vi "main_RL.vi"() -> ()   [LabVIEW 2017]
panel:
  in  "Tab Control":enum32{"Page 1", "Page 2"}(tab)
  in  "Next Button":bool
  out "Heater ON/OFF":bool caption="Heater"
  out "Pump ON/OFF":bool caption="Pump"
  in  "F1_F3":bool
  in  "T1_T3":bool
  out "NI1":tag caption="NI device"
  in  "Exit":bool
  in  "Tab Control 4":enum32{"Charts", "Diagram"}(tab)
  in  "Save as image 6":bool
  in  "Save as Excel 6":bool
  in  "Pause Button 6":bool
  in  "Reset Chart 6":bool
  in  "Save as image 5":bool
  in  "Save as Excel 5":bool
  in  "Pause Button 5":bool
  in  "Reset Chart 5":bool
  in  "Tab Control 2":enum32{"Page 1", "Page 2"}(tab)
  in  "Save as image 3":bool
  in  "Save as Excel 3":bool
  in  "Pause Button 3":bool
  in  "Reset Chart 3":bool
  out "T1 chart":dbl(graph)
  in  "Reset Chart":bool
  in  "Pause Button":bool
  in  "Save as Excel":bool
  in  "Save as image":bool
  out "T3 chart":dbl(graph)
  out "T2 chart":dbl(graph)
  out "F2 chart":dbl(graph)
  in  "Tab Control 3":enum32{"Page 1", "Page 2"}(tab)
  in  "Reset Chart 4":bool
  in  "Pause Button 4":bool
  in  "Save as Excel 4":bool
  in  "Save as image 4":bool
  out "F1 chart":dbl(graph)
  in  "Reset Chart 2":bool
  in  "Pause Button 2":bool
  in  "Save as Excel 2":bool
  in  "Save as image 2":bool
  out "F3 chart":dbl(graph)
  out "Heater":bool
  out "FlowMeter 3":bool
  out "FlowMeter 2":bool
  out "Pump":bool
  out "FlowMeter":bool
  out "T1":dbl format="%#.3f"
  out "T3":dbl format="%#_3f"
  out "F1":dbl format="%#.3f"
  out "F3":dbl format="%#_3f"
  out "T2":dbl format="%#.3f"
  out "F2":dbl format="%#.3f"
  in  "Pump 2":bool
  in  "Heater ON/OFF 2":bool
  # "Recycle Loops Unit"
  # "Cold Water Supply"
  # "To Drain"
  # "Water Heater"
  # "Water Filter"
  # "Pressure reducing valve"
  # "Pump"
  # "Throttling Valve"
  # "Temperature Sensor\n(T2)"
  # "Flow meter\n(F3)"
  # "Flow meter\n(F1)"
  # "Flow meter\n(F2)"
  # "Temperature Sensor\n(T1)"
  # "Temperature Sensor\n(T3)"
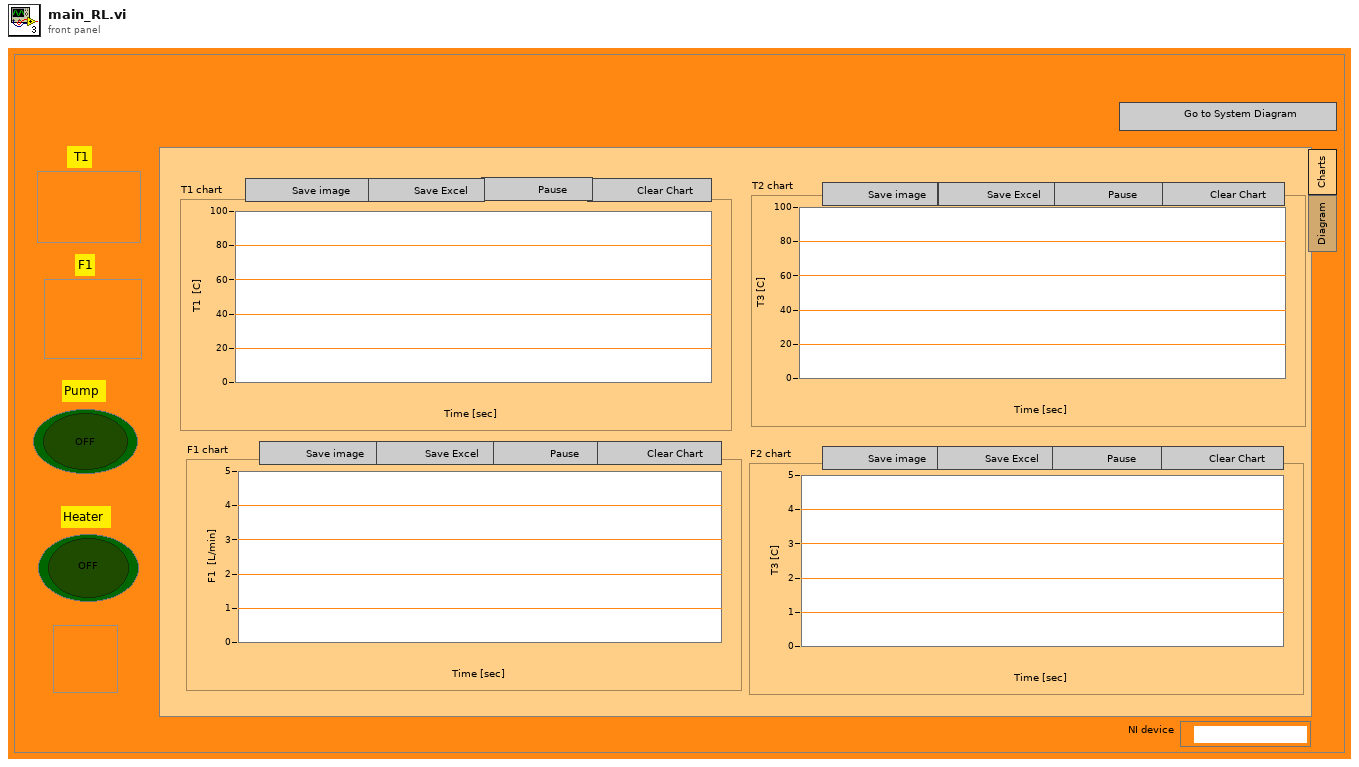
[diagram p1: front panel]
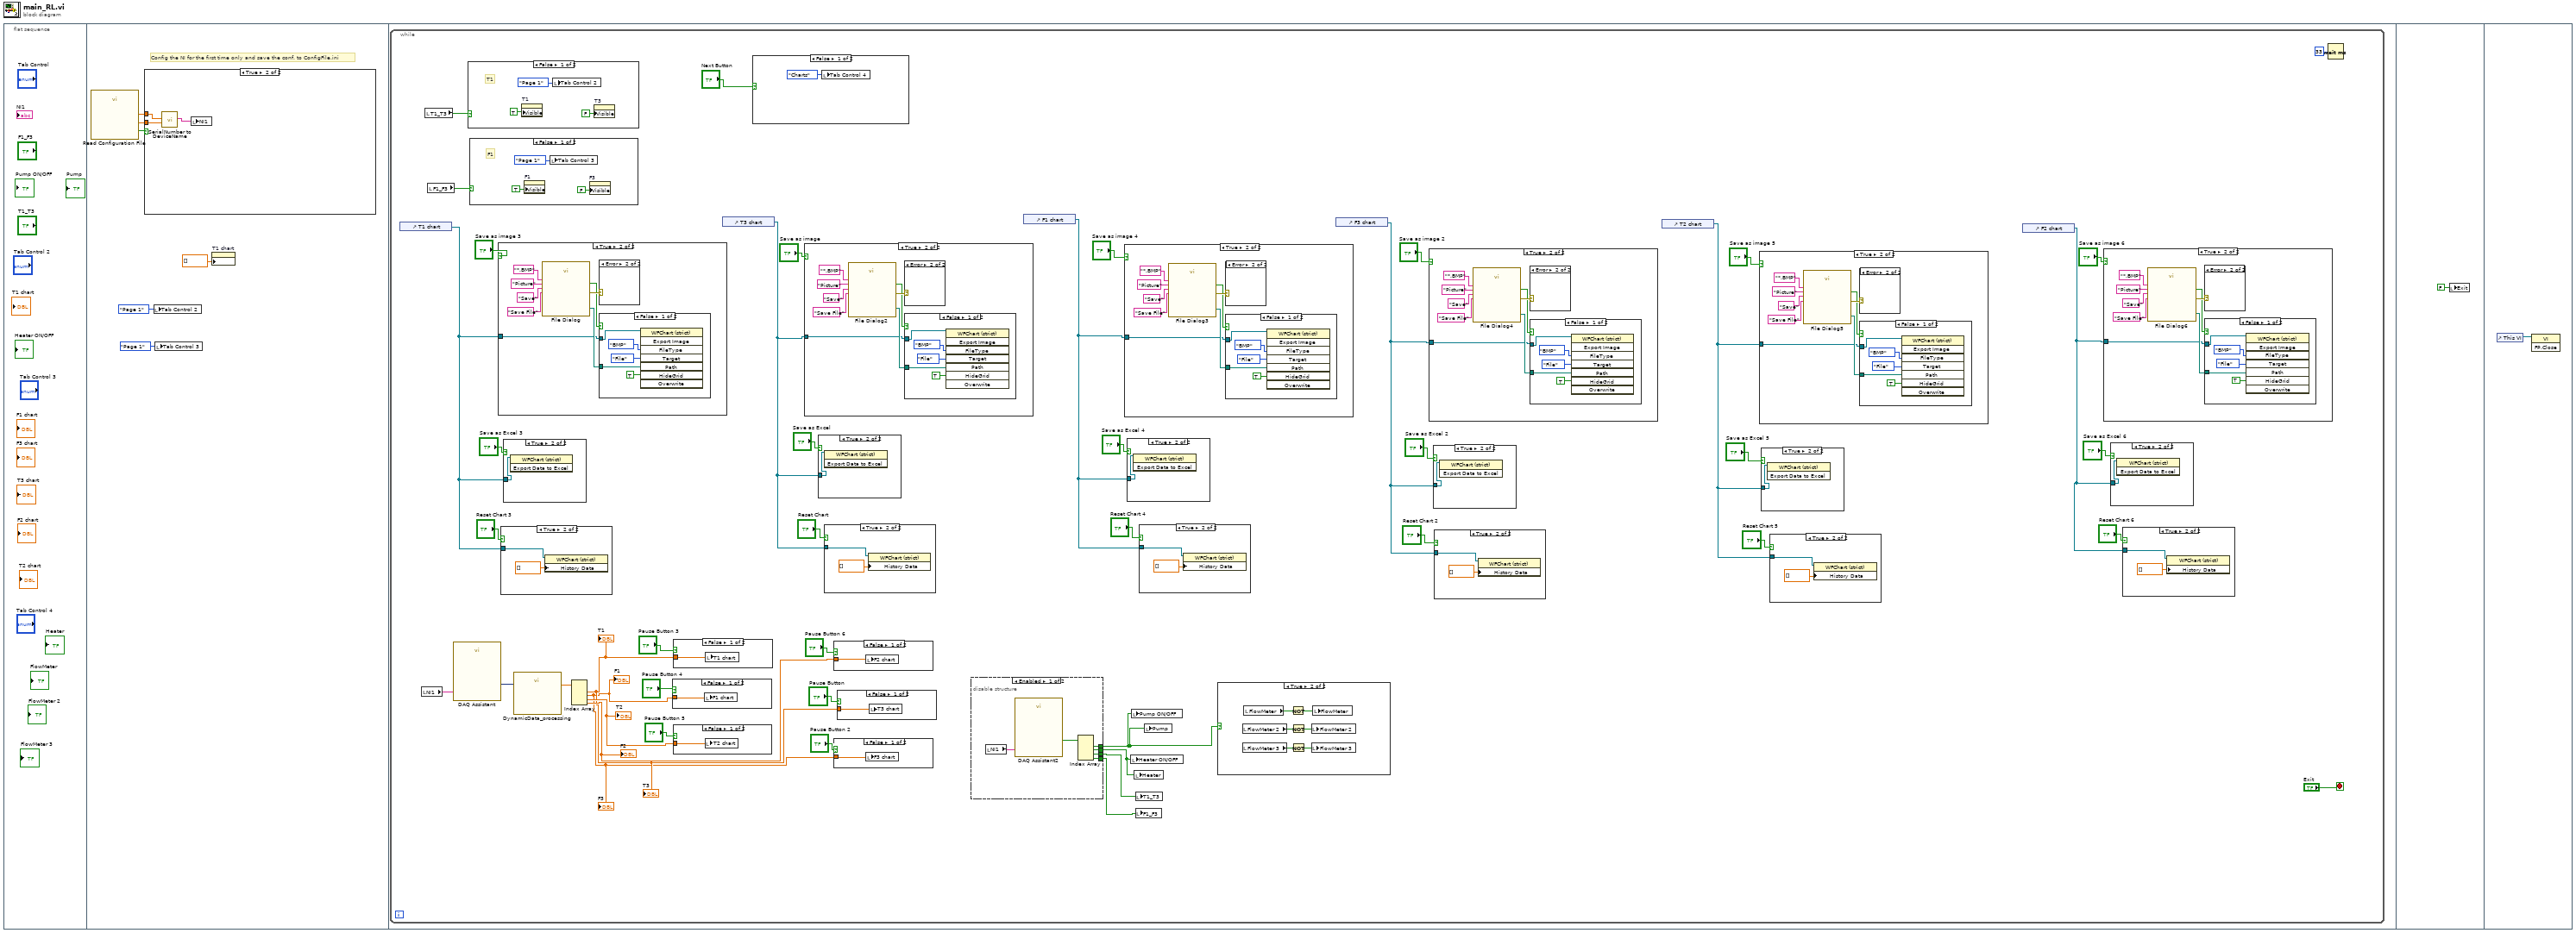
[diagram p0: block diagram]
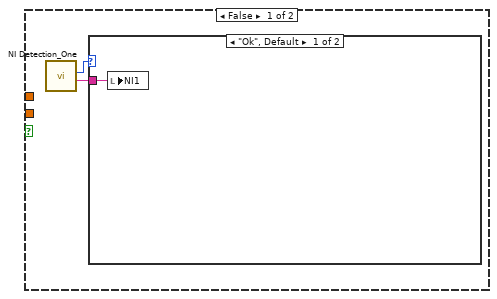
[diagram p2: hidden frame]
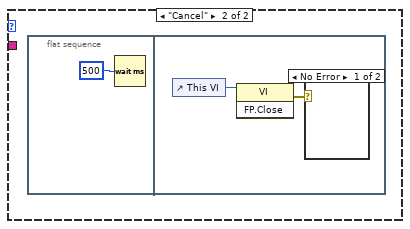
[diagram p3: hidden frame]
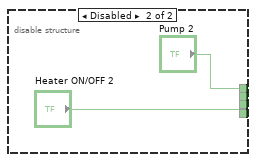
[diagram p5: hidden frame]
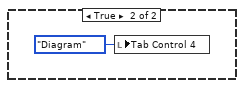
[diagram p7: hidden frame]
diagram:
  n1 = flat-sequence {
    frame #0 {
    }
    frame #1 {
      # "Config the NI for the first time only and save the conf. to ConfigFile.ini"
      n2 = call "Read Configuration File.vi"() -> ("Serial Numbers Found"=w2:bool, "NI1"=w3:dbl, "NI2"=w4:dbl)  [unwired: 13 in]
      n3 = case shown="True" w2 {
        tunnel: w3 -> [_ w15]
        tunnel: w4 -> [_ w14]
        frame False {
          n4 = call "NI Detection_One.vi"() -> ("NI 1"=w7:tag, "Ok/Cancel"=w8:enum16{"Ok", "Cancel"})  [unwired: 8 in, 1 out]
          n5 = case shown="\"Ok\", Default" w8 {
            tunnel: w7 -> [w9 _]
            frame "Ok", Default {
              n6 = local write "NI1"(w9) -> ()
            }
            frame "Cancel" {
              n7 = flat-sequence {
                frame #0 {
                  n8 = Wait (ms)(milliseconds to wait=u32 500) -> ()  [unwired: 1 out]
                }
                frame #1 {
                  n9 = control-ref of="This VI"() -> (w12:refnum<vi>)
                  n10 = invoke class="VI" method="FP.Close"(reference=w12) -> (error out=w11:errorcluster)  [unwired: 2 in, 2 out]
                  n11 = case shown="No Error" w11 {
                    frame No Error {
                    }
                    frame Error {
                    }
                  }
                }
              }
            }
          }
        }
        frame True {
          n12 = call "SerialNumber to DeviceName.vi"("NI2 Serial Number"=w14, "NI1 Serial Number"=w15) -> ("NI1 Device Name"=w13:tag)  [unwired: 8 in, 1 out]
          n13 = local write "NI1"(w13) -> ()
        }
      }
      n14 = local write "Tab Control 2"(enum32{"Page 1", "Page 2"}."Page 1" ("Tab Control 2")) -> ()
      n15 = local write "Tab Control 3"(enum32{"Page 1", "Page 2"}."Page 1" ("Tab Control 2")) -> ()
      n16 = property on="T1 chart" class="WFChart (strict)"("History Data"=dbl[] []) -> ()  [unwired: 2 in, 2 out]
    }
    frame #2 {
      n17 = while {
        stop <- "Exit" stop-if-true
        n18 = control-ref of="T1 chart"() -> (w54:refnum<vi>)
        n19 = local read "NI1"() -> (w32:tag)
        n20 = local read "T1_T3"() -> (w60:bool)
        n21 = local read "F1_F3"() -> (w59:bool)
        n22 = call "DAQ Assistant"("device name"=w32) -> ("data"=w33:dynamicdata)  [unwired: 16 in, 2 out]
        n23 = case shown="False" w60 {
          frame False {
            # "T1"
            n24 = property on="T1" class="DigNum (strict)"("Visible"=TRUE) -> ()  [unwired: 2 in, 2 out]
            n25 = local write "Tab Control 2"(enum32{"Page 1", "Page 2"}."Page 1" ("Tab Control 2")) -> ()
            n26 = property on="T3" class="DigNum (strict)"("Visible"=FALSE) -> ()  [unwired: 2 in, 2 out]
          }
          frame True {
            # "T3"
            n27 = property on="T1" class="DigNum (strict)"("Visible"=FALSE) -> ()  [unwired: 2 in, 2 out]
            n28 = local write "Tab Control 2"(enum32{"Page 1", "Page 2"}."Page 2" ("Tab Control 2")) -> ()
            n29 = property on="T3" class="DigNum (strict)"("Visible"=TRUE) -> ()  [unwired: 2 in, 2 out]
          }
        }
        n30 = case shown="False" w59 {
          frame False {
            # "F1"
            n31 = property on="F1" class="DigNum (strict)"("Visible"=TRUE) -> ()  [unwired: 2 in, 2 out]
            n32 = local write "Tab Control 3"(enum32{"Page 1", "Page 2"}."Page 1" ("Tab Control 2")) -> ()
            n33 = property on="F3" class="DigNum (strict)"("Visible"=FALSE) -> ()  [unwired: 2 in, 2 out]
          }
          frame True {
            # "F3"
            n34 = property on="F1" class="DigNum (strict)"("Visible"=FALSE) -> ()  [unwired: 2 in, 2 out]
            n35 = local write "Tab Control 3"(enum32{"Page 1", "Page 2"}."Page 2" ("Tab Control 2")) -> ()
            n36 = property on="F3" class="DigNum (strict)"("Visible"=TRUE) -> ()  [unwired: 2 in, 2 out]
          }
        }
        n37 = case shown="True" "Save as image 3" {
          tunnel: w54 -> [_ w167]
          frame False {
          }
          frame True {
            n38 = call "File Dialog"("prompt"="Save File", "button label"="Save", "pattern (all files)"="*.BMP", "pattern label"="Picture") -> ("selected path"=w169:path, "cancelled"=w168:bool, "error out"=w170:errorcluster)  [unwired: 8 in, 1 out]
            n39 = case shown="Error" w170 {
              frame No Error {
              }
              frame Error {
              }
            }
            n40 = case shown="False" w168 {
              tunnel: w169 -> [w177 _]
              tunnel: w167 -> [w175 _]
              frame False {
                n41 = invoke on="Invoke Node" class="WFChart (strict)" method="Export Image"(reference=w175, "FileType"=enum32{"BMP", "EPS", "EMF", "PICT"}."BMP" ("File Type"), "Target"=enum32{"File", "Clipboard"}."File", "Path"=w177, "HideGrid"=TRUE ("Hide Grid")) -> ()  [unwired: 3 in, 8 out]
              }
              frame True {
              }
            }
          }
        }
        n42 = case shown="True" "Reset Chart 3" {
          tunnel: w54 -> [_ w165]
          frame False {
          }
          frame True {
            n43 = property on="Property Node" class="WFChart (strict)"(reference=w165, "History Data"=dbl[] []) -> ()  [unwired: 1 in, 2 out]
          }
        }
        n44 = case shown="True" "Save as Excel 3" {
          tunnel: w54 -> [_ w166]
          frame False {
          }
          frame True {
            n45 = invoke on="Invoke Node" class="WFChart (strict)" method="Export Data to Excel"(reference=w166) -> ()  [unwired: 2 in, 3 out]
          }
        }
        n46 = call "DynamicData_processing.vi"("data"=w33) -> ("DATA"=w34:dbl[])
        n47 = Index Array(array=w34) -> (element #1=w19:dbl, element #2=w18:dbl, element #3=w28:dbl, element #4=w26:dbl)  [unwired: 4 in]
        "T1" <- w19
        "F1" <- w18
        "T2" <- w28
        "F2" <- w26
        "T3" <- w19
        "F3" <- w18
        n48 = case shown="False" "Pause Button 4" {
          tunnel: w18 -> [w81 _]
          frame False {
            n49 = local write "F1 chart"(w81) -> ()
          }
          frame True {
          }
        }
        n50 = case shown="False" "Pause Button 5" {
          tunnel: w28 -> [w82 _]
          frame False {
            n51 = local write "T2 chart"(w82) -> ()
          }
          frame True {
          }
        }
        n52 = case shown="False" "Pause Button 3" {
          tunnel: w19 -> [w83 _]
          frame False {
            n53 = local write "T1 chart"(w83) -> ()
          }
          frame True {
          }
        }
        n54 = control-ref of="T3 chart"() -> (w50:refnum<vi>)
        n55 = case shown="False" "Next Button" {
          frame False {
            n56 = local write "Tab Control 4"(enum32{"Charts", "Diagram"}."Charts" ("Tab Control 4")) -> ()
          }
          frame True {
            n57 = local write "Tab Control 4"(enum32{"Charts", "Diagram"}."Diagram" ("Tab Control 4")) -> ()
          }
        }
        n58 = case shown="True" "Save as image" {
          tunnel: w50 -> [_ w151]
          frame False {
          }
          frame True {
            n59 = call "File Dialog2"("prompt"="Save File", "button label"="Save", "pattern (all files)"="*.BMP", "pattern label"="Picture") -> ("selected path"=w153:path, "cancelled"=w152:bool, "error out"=w154:errorcluster)  [unwired: 8 in, 1 out]
            n60 = case shown="Error" w154 {
              frame No Error {
              }
              frame Error {
              }
            }
            n61 = case shown="False" w152 {
              tunnel: w153 -> [w161 _]
              tunnel: w151 -> [w159 _]
              frame False {
                n62 = invoke on="Invoke Node" class="WFChart (strict)" method="Export Image"(reference=w159, "FileType"=enum32{"BMP", "EPS", "EMF", "PICT"}."BMP" ("File Type"), "Target"=enum32{"File", "Clipboard"}."File", "Path"=w161, "HideGrid"=TRUE ("Hide Grid")) -> ()  [unwired: 3 in, 8 out]
              }
              frame True {
              }
            }
          }
        }
        n63 = case shown="True" "Save as Excel" {
          tunnel: w50 -> [_ w150]
          frame False {
          }
          frame True {
            n64 = invoke on="Invoke Node" class="WFChart (strict)" method="Export Data to Excel"(reference=w150) -> ()  [unwired: 2 in, 3 out]
          }
        }
        n65 = case shown="True" "Reset Chart" {
          tunnel: w50 -> [_ w149]
          frame False {
          }
          frame True {
            n66 = property on="Property Node" class="WFChart (strict)"(reference=w149, "History Data"=dbl[] []) -> ()  [unwired: 1 in, 2 out]
          }
        }
        n67 = case shown="False" "Pause Button 6" {
          tunnel: w26 -> [w80 _]
          frame False {
            n68 = local write "F2 chart"(w80) -> ()
          }
          frame True {
          }
        }
        n69 = case shown="False" "Pause Button 2" {
          tunnel: w18 -> [w78 _]
          frame False {
            n70 = local write "F3 chart"(w78) -> ()
          }
          frame True {
          }
        }
        n71 = case shown="False" "Pause Button" {
          tunnel: w19 -> [w79 _]
          frame False {
            n72 = local write "T3 chart"(w79) -> ()
          }
          frame True {
          }
        }
        n73 = disable-structure shown="Enabled" {
          disable-tunnel: [w65 "Heater ON/OFF 2"] -> w20
          disable-tunnel: [w64 "Pump 2"] -> w21
          disable-tunnel: [w63 _] -> w17
          disable-tunnel: [w62 _] -> w16
          frame Enabled {
            n74 = local read "NI1"() -> (w67:tag)
            n75 = call "DAQ Assistant2"("device name"=w67) -> ("data"=w66:bool[])  [unwired: 16 in, 2 out]
            n76 = Index Array(array=w66) -> (element #1=w64:bool, element #2=w65:bool, element #3=w63:bool, element #4=w62:bool)  [unwired: 4 in]
          }
          frame Disabled {
          }
        }
        n77 = control-ref of="F1 chart"() -> (w46:refnum<vi>)
        n78 = case shown="True" "Save as image 4" {
          tunnel: w46 -> [_ w135]
          frame False {
          }
          frame True {
            n79 = call "File Dialog3"("prompt"="Save File", "button label"="Save", "pattern (all files)"="*.BMP", "pattern label"="Picture") -> ("selected path"=w137:path, "cancelled"=w136:bool, "error out"=w138:errorcluster)  [unwired: 8 in, 1 out]
            n80 = case shown="Error" w138 {
              frame No Error {
              }
              frame Error {
              }
            }
            n81 = case shown="False" w136 {
              tunnel: w137 -> [w145 _]
              tunnel: w135 -> [w143 _]
              frame False {
                n82 = invoke on="Invoke Node" class="WFChart (strict)" method="Export Image"(reference=w143, "FileType"=enum32{"BMP", "EPS", "EMF", "PICT"}."BMP" ("File Type"), "Target"=enum32{"File", "Clipboard"}."File", "Path"=w145, "HideGrid"=TRUE ("Hide Grid")) -> ()  [unwired: 3 in, 8 out]
              }
              frame True {
              }
            }
          }
        }
        n83 = case shown="True" "Save as Excel 4" {
          tunnel: w46 -> [_ w134]
          frame False {
          }
          frame True {
            n84 = invoke on="Invoke Node" class="WFChart (strict)" method="Export Data to Excel"(reference=w134) -> ()  [unwired: 2 in, 3 out]
          }
        }
        n85 = local write "Heater ON/OFF"(w20) -> ()
        n86 = local write "Pump ON/OFF"(w21) -> ()
        n87 = local write "Heater"(w20) -> ()
        n88 = local write "T1_T3"(w17) -> ()
        n89 = local write "F1_F3"(w16) -> ()
        n90 = case shown="True" "Reset Chart 4" {
          tunnel: w46 -> [_ w133]
          frame False {
          }
          frame True {
            n91 = property on="Property Node" class="WFChart (strict)"(reference=w133, "History Data"=dbl[] []) -> ()  [unwired: 1 in, 2 out]
          }
        }
        n92 = local write "Pump"(w21) -> ()
        n93 = case shown="True" w21 {
          frame False {
          }
          frame True {
            n94 = local read "FlowMeter 2"() -> (w73:bool)
            n95 = local read "FlowMeter 3"() -> (w70:bool)
            n96 = local read "FlowMeter"() -> (w74:bool)
            n97 = Not(x=w74) -> (.not. x?=w75:bool)
            n98 = Not(x=w73) -> (.not. x?=w72:bool)
            n99 = Not(x=w70) -> (.not. x?=w71:bool)
            n100 = local write "FlowMeter 2"(w72) -> ()
            n101 = local write "FlowMeter 3"(w71) -> ()
            n102 = local write "FlowMeter"(w75) -> ()
          }
        }
        n103 = control-ref of="F3 chart"() -> (w42:refnum<vi>)
        n104 = case shown="True" "Save as image 2" {
          tunnel: w42 -> [_ w119]
          frame False {
          }
          frame True {
            n105 = call "File Dialog4"("prompt"="Save File", "button label"="Save", "pattern (all files)"="*.BMP", "pattern label"="Picture") -> ("selected path"=w121:path, "cancelled"=w120:bool, "error out"=w122:errorcluster)  [unwired: 8 in, 1 out]
            n106 = case shown="Error" w122 {
              frame No Error {
              }
              frame Error {
              }
            }
            n107 = case shown="False" w120 {
              tunnel: w121 -> [w129 _]
              tunnel: w119 -> [w127 _]
              frame False {
                n108 = invoke on="Invoke Node" class="WFChart (strict)" method="Export Image"(reference=w127, "FileType"=enum32{"BMP", "EPS", "EMF", "PICT"}."BMP" ("File Type"), "Target"=enum32{"File", "Clipboard"}."File", "Path"=w129, "HideGrid"=TRUE ("Hide Grid")) -> ()  [unwired: 3 in, 8 out]
              }
              frame True {
              }
            }
          }
        }
        n109 = case shown="True" "Save as Excel 2" {
          tunnel: w42 -> [_ w118]
          frame False {
          }
          frame True {
            n110 = invoke on="Invoke Node" class="WFChart (strict)" method="Export Data to Excel"(reference=w118) -> ()  [unwired: 2 in, 3 out]
          }
        }
        n111 = case shown="True" "Reset Chart 2" {
          tunnel: w42 -> [_ w117]
          frame False {
          }
          frame True {
            n112 = property on="Property Node" class="WFChart (strict)"(reference=w117, "History Data"=dbl[] []) -> ()  [unwired: 1 in, 2 out]
          }
        }
        n113 = control-ref of="T2 chart"() -> (w38:refnum<vi>)
        n114 = case shown="True" "Save as image 5" {
          tunnel: w38 -> [_ w103]
          frame False {
          }
          frame True {
            n115 = call "File Dialog5"("prompt"="Save File", "button label"="Save", "pattern (all files)"="*.BMP", "pattern label"="Picture") -> ("selected path"=w105:path, "cancelled"=w104:bool, "error out"=w106:errorcluster)  [unwired: 8 in, 1 out]
            n116 = case shown="Error" w106 {
              frame No Error {
              }
              frame Error {
              }
            }
            n117 = case shown="False" w104 {
              tunnel: w105 -> [w113 _]
              tunnel: w103 -> [w111 _]
              frame False {
                n118 = invoke on="Invoke Node" class="WFChart (strict)" method="Export Image"(reference=w111, "FileType"=enum32{"BMP", "EPS", "EMF", "PICT"}."BMP" ("File Type"), "Target"=enum32{"File", "Clipboard"}."File", "Path"=w113, "HideGrid"=TRUE ("Hide Grid")) -> ()  [unwired: 3 in, 8 out]
              }
              frame True {
              }
            }
          }
        }
        n119 = case shown="True" "Save as Excel 5" {
          tunnel: w38 -> [_ w102]
          frame False {
          }
          frame True {
            n120 = invoke on="Invoke Node" class="WFChart (strict)" method="Export Data to Excel"(reference=w102) -> ()  [unwired: 2 in, 3 out]
          }
        }
        n121 = case shown="True" "Reset Chart 5" {
          tunnel: w38 -> [_ w101]
          frame False {
          }
          frame True {
            n122 = property on="Property Node" class="WFChart (strict)"(reference=w101, "History Data"=dbl[] []) -> ()  [unwired: 1 in, 2 out]
          }
        }
        n123 = control-ref of="F2 chart"() -> (w35:refnum<vi>)
        n124 = case shown="True" "Save as image 6" {
          tunnel: w35 -> [_ w87]
          frame False {
          }
          frame True {
            n125 = call "File Dialog6"("prompt"="Save File", "button label"="Save", "pattern (all files)"="*.BMP", "pattern label"="Picture") -> ("selected path"=w89:path, "cancelled"=w88:bool, "error out"=w90:errorcluster)  [unwired: 8 in, 1 out]
            n126 = case shown="Error" w90 {
              frame No Error {
              }
              frame Error {
              }
            }
            n127 = case shown="False" w88 {
              tunnel: w89 -> [w97 _]
              tunnel: w87 -> [w95 _]
              frame False {
                n128 = invoke on="Invoke Node" class="WFChart (strict)" method="Export Image"(reference=w95, "FileType"=enum32{"BMP", "EPS", "EMF", "PICT"}."BMP" ("File Type"), "Target"=enum32{"File", "Clipboard"}."File", "Path"=w97, "HideGrid"=TRUE ("Hide Grid")) -> ()  [unwired: 3 in, 8 out]
              }
              frame True {
              }
            }
          }
        }
        n129 = case shown="True" "Save as Excel 6" {
          tunnel: w35 -> [_ w86]
          frame False {
          }
          frame True {
            n130 = invoke on="Invoke Node" class="WFChart (strict)" method="Export Data to Excel"(reference=w86) -> ()  [unwired: 2 in, 3 out]
          }
        }
        n131 = case shown="True" "Reset Chart 6" {
          tunnel: w35 -> [_ w85]
          frame False {
          }
          frame True {
            n132 = property on="Property Node" class="WFChart (strict)"(reference=w85, "History Data"=dbl[] []) -> ()  [unwired: 1 in, 2 out]
          }
        }
        n133 = Wait (ms)(milliseconds to wait=u32 33) -> ()  [unwired: 1 out]
      }
    }
    frame #3 {
      n134 = local write "Exit"(FALSE ("Exit")) -> ()
    }
    frame #4 {
      n135 = control-ref of="This VI"() -> (w193:refnum<vi>)
      n136 = invoke class="VI" method="FP.Close"(reference=w193) -> ()  [unwired: 2 in, 3 out]
    }
  }
